vi "ke37xx Read Measurement Buffer.vi"(0 "VISA Resource Name":refnum<visa-resource-name>, 1 "Data To Read (All)":T1={"Readings"=TRUE, "Time Stamps"=TRUE, "Channels"=TRUE, "Units"=TRUE}, 5 "Buffer Name":string, 7 "Start Index (1)":i32=1 min=1, 9 "End Index (-1: Read All)":i32=-1 min=-1, 11 "error in (no error)":errorcluster, 12 "Time Stamp Format (0: UTC)":enum16{"UTC Time", "1588 Time"}(ring), 13 "Bytes To Read (1024)":u32=1024, 14 "Timeout (10 seconds)":u32=10000) -> (2 "Units":string[](array[string]), 3 "Channels":string[](array[string]), 4 "VISA Resource Name Out":refnum<visa-resource-name>, 6 "Readings":dbl[](array[numeric]) format="%#_6e", 8 "Time Stamps":cluster{"Seconds":u32, "Fraction":dbl}[](array[cluster]), 10 "Base Time Stamp":cluster{"Seconds":u32, "Fraction":dbl}, 15 "error out":errorcluster)   [LabVIEW 2009, in "Keithley 3700 Series.lvlib"]
doc: "This VI allows you to retrieve readings stored in a measurement buffer. You can optionally retrieve timestamp data, formatted readigns, measurement units, and channels measured."
uses:
  <instrlib>/Keithley 3706/Keithley 3700 Series.lvlib
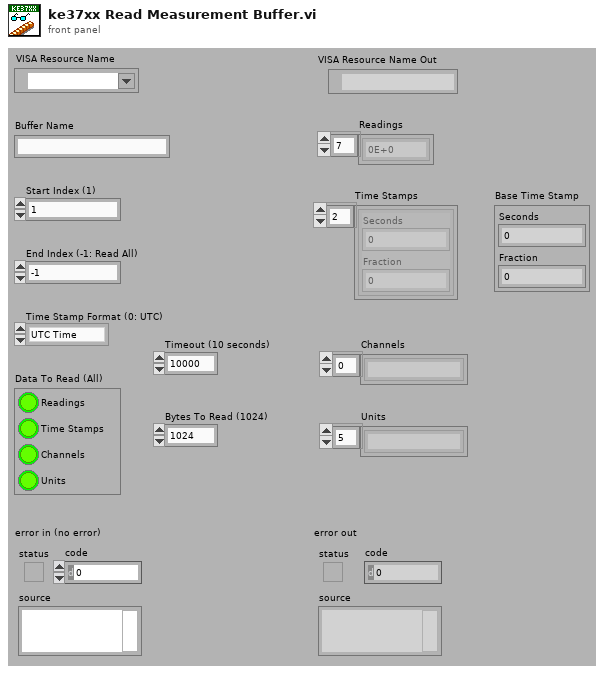
[diagram p1: front panel]
types:
  T1 = cluster{"Readings":bool, "Time Stamps":bool, "Channels":bool, "Units":bool}
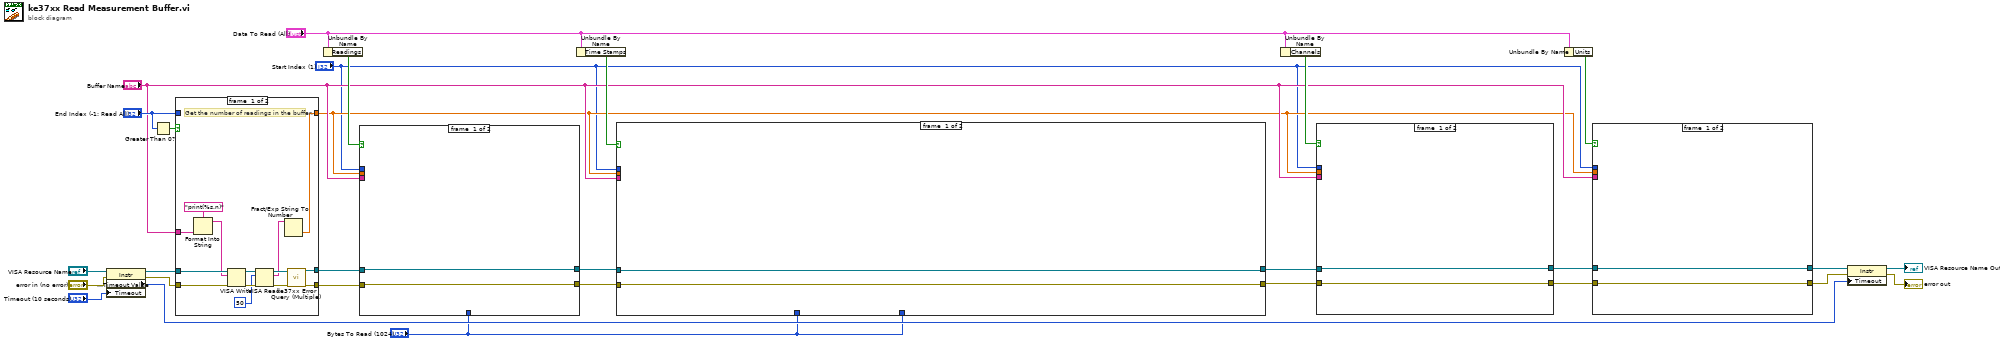
[diagram p0: block diagram]
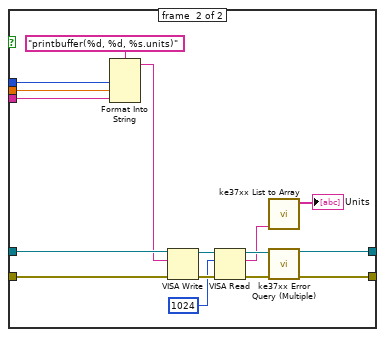
[diagram p2: hidden frame]
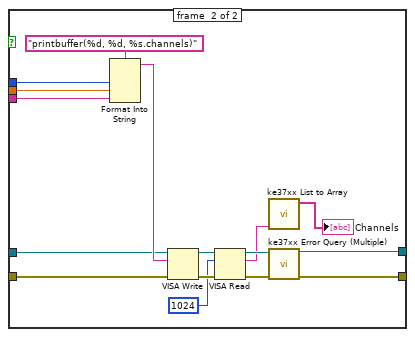
[diagram p3: hidden frame]
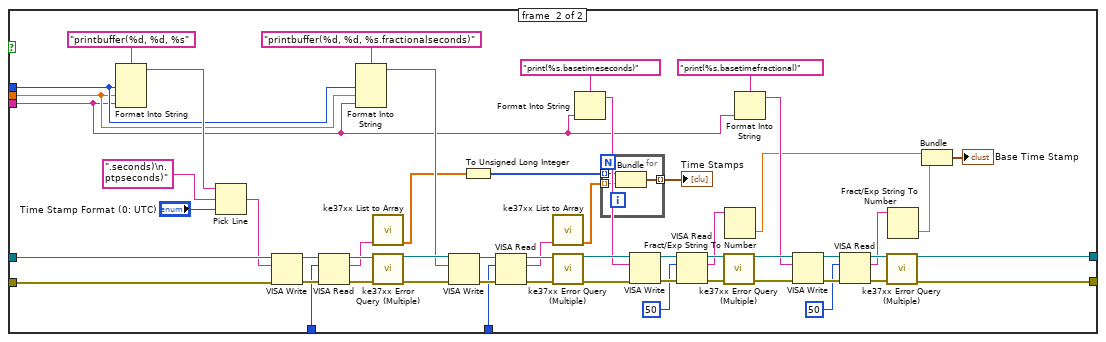
[diagram p4: hidden frame]
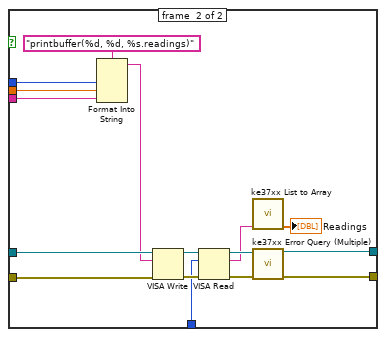
[diagram p5: hidden frame]
diagram:
  n1 = property class="Instr"(reference="VISA Resource Name", error in="error in (no error)", "Timeout"="Timeout (10 seconds)") -> (reference out=w12:refnum<visa-resource-name>, error out=w8:errorcluster, "General Settings:Timeout Value"=w2:u32)
  n2 = Greater Than 0?(x="End Index (-1: Read All)") -> (x > 0?=w29:bool)
  n3 = case shown="False" w29 {
    tunnel: w12 -> [w43 w45]
    tunnel: w8 -> [w42 w44]
    tunnel: [w41 w45] -> w28
    tunnel: [w40 w44] -> w27
    tunnel: "End Index (-1: Read All)" -> [_ w46]
    tunnel: [w31 w46] -> w15
    tunnel: "Buffer Name" -> [w30 _]
    frame #0 {
      # "Get the number of readings in the buffer."
      n4 = Format Into String(format string="print(%s.n)", w30) -> (resulting string=w38:string)  [unwired: 2 in, 1 out]
      n5 = VISA Write(VISA resource name=w43, write buffer=w38, error in (no error)=w42) -> (VISA resource name out=w37:refnum<visa-resource-name>, error out=w35:errorcluster)  [unwired: 1 out]
      n6 = VISA Read(VISA resource name=w37, byte count=u32 50, error in (no error)=w35) -> (VISA resource name out=w36:refnum<visa-resource-name>, read buffer=w32:string, error out=w34:errorcluster)  [unwired: 1 out]
      n7 = Fract/Exp String To Number(string=w32) -> (number=w31:dbl)  [unwired: 4 out]
      n8 = call <instrlib>:"ke37xx Error Query (Multiple).vi"("VISA resource name"=w36, "error in (no error)"=w34) -> ("VISA resource name out"=w41:refnum<visa-resource-name>, "error out"=w40:errorcluster)  [unwired: 12 out]
    }
    frame #1 {
    }
  }
  n9 = Unbundle By Name("Data To Read (All)") -> ("Readings"=w26:bool)
  n10 = case shown="True" w26 {
    tunnel: "Start Index (1)" -> [_ w62]
    tunnel: w28 -> [w48 w58]
    tunnel: w27 -> [w47 w57]
    tunnel: [w48 w56] -> w25
    tunnel: [w47 w55] -> w24
    tunnel: w15 -> [_ w52]
    tunnel: "Buffer Name" -> [_ w51]
    tunnel: "Bytes To Read (1024)" -> [_ w49]
    frame #0 {
    }
    frame #1 {
      n11 = Format Into String(format string="printbuffer(%d, %d, %s.readings)", w62, w52, w51) -> (resulting string=w54:string)  [unwired: 2 in, 1 out]
      n12 = VISA Write(VISA resource name=w58, write buffer=w54, error in (no error)=w57) -> (VISA resource name out=w59:refnum<visa-resource-name>, error out=w64:errorcluster)  [unwired: 1 out]
      n13 = VISA Read(VISA resource name=w59, byte count=w49, error in (no error)=w64) -> (VISA resource name out=w60:refnum<visa-resource-name>, read buffer=w50:string, error out=w61:errorcluster)  [unwired: 1 out]
      n14 = call <instrlib>:"ke37xx List to Array.vi"("List"=w50) -> ("Output Number Array"=→"Readings":dbl[])  [unwired: 1 in, 5 out]
      n15 = call <instrlib>:"ke37xx Error Query (Multiple).vi"("VISA resource name"=w60, "error in (no error)"=w61) -> ("VISA resource name out"=w56:refnum<visa-resource-name>, "error out"=w55:errorcluster)  [unwired: 12 out]
    }
  }
  n16 = Unbundle By Name("Data To Read (All)") -> ("Time Stamps"=w23:bool)
  n17 = case shown="True" w23 {
    tunnel: "Start Index (1)" -> [_ w104]
    tunnel: w25 -> [w66 w115]
    tunnel: w24 -> [w65 w114]
    tunnel: w15 -> [_ w103]
    tunnel: "Buffer Name" -> [_ w88]
    tunnel: [w66 w79] -> w11
    tunnel: [w65 w78] -> w10
    tunnel: "Bytes To Read (1024)" -> [_ w68]
    tunnel: "Bytes To Read (1024)" -> [_ w67]
    frame #0 {
    }
    frame #1 {
      n18 = Format Into String(format string="printbuffer(%d, %d, %s", w104, w103, w88) -> (resulting string=w111:string)  [unwired: 2 in, 1 out]
      n19 = Pick Line(string ("")=w111, multi-line string=".seconds)\n.ptpseconds)", line index="Time Stamp Format (0: UTC)") -> (output string=w110:string)
      n20 = VISA Write(VISA resource name=w115, write buffer=w110, error in (no error)=w114) -> (VISA resource name out=w116:refnum<visa-resource-name>, error out=w120:errorcluster)  [unwired: 1 out]
      n21 = VISA Read(VISA resource name=w116, byte count=w68, error in (no error)=w120) -> (VISA resource name out=w117:refnum<visa-resource-name>, read buffer=w77:string, error out=w118:errorcluster)  [unwired: 1 out]
      n22 = Format Into String(format string="printbuffer(%d, %d, %s.fractionalseconds)", w104, w103, w88) -> (resulting string=w102:string)  [unwired: 2 in, 1 out]
      n23 = call <instrlib>:"ke37xx List to Array.vi"("List"=w77) -> ("Output Number Array"=w72:dbl[])  [unwired: 1 in, 5 out]
      n24 = call <instrlib>:"ke37xx Error Query (Multiple).vi"("VISA resource name"=w117, "error in (no error)"=w118) -> ("VISA resource name out"=w107:refnum<visa-resource-name>, "error out"=w106:errorcluster)  [unwired: 12 out]
      n25 = VISA Write(VISA resource name=w107, write buffer=w102, error in (no error)=w106) -> (VISA resource name out=w109:refnum<visa-resource-name>, error out=w108:errorcluster)  [unwired: 1 out]
      n26 = To Unsigned Long Integer(number=w72) -> (unsigned 32bit integer=w71:u32[])
      n27 = VISA Read(VISA resource name=w109, byte count=w67, error in (no error)=w108) -> (VISA resource name out=w96:refnum<visa-resource-name>, read buffer=w76:string, error out=w95:errorcluster)  [unwired: 1 out]
      n28 = call <instrlib>:"ke37xx List to Array.vi"("List"=w76) -> ("Output Number Array"=w70:dbl[])  [unwired: 1 in, 5 out]
      n29 = call <instrlib>:"ke37xx Error Query (Multiple).vi"("VISA resource name"=w96, "error in (no error)"=w95) -> ("VISA resource name out"=w94:refnum<visa-resource-name>, "error out"=w93:errorcluster)  [unwired: 12 out]
      n30 = Format Into String(format string="print(%s.basetimeseconds)", w88) -> (resulting string=w90:string)  [unwired: 2 in, 1 out]
      n31 = for {
        tunnel: w71 -> [w124] mode=indexing
        tunnel: w70 -> [w123] mode=indexing
        tunnel: [w122] -> w69 mode=indexing
        n32 = Bundle(w124, w123) -> (w122:cluster{u32, dbl})  [unwired: 1 out]
      }
      "Time Stamps" <- w69
      n33 = VISA Write(VISA resource name=w94, write buffer=w90, error in (no error)=w93) -> (VISA resource name out=w99:refnum<visa-resource-name>, error out=w101:errorcluster)  [unwired: 1 out]
      n34 = VISA Read(VISA resource name=w99, byte count=u32 50, error in (no error)=w101) -> (VISA resource name out=w92:refnum<visa-resource-name>, read buffer=w89:string, error out=w91:errorcluster)  [unwired: 1 out]
      n35 = call <instrlib>:"ke37xx Error Query (Multiple).vi"("VISA resource name"=w92, "error in (no error)"=w91) -> ("VISA resource name out"=w83:refnum<visa-resource-name>, "error out"=w82:errorcluster)  [unwired: 12 out]
      n36 = Fract/Exp String To Number(string=w89) -> (number=w75:dbl)  [unwired: 1 in, 3 out]
      n37 = Format Into String(format string="print(%s.basetimefractional)", w88) -> (resulting string=w81:string)  [unwired: 2 in, 1 out]
      n38 = VISA Write(VISA resource name=w83, write buffer=w81, error in (no error)=w82) -> (VISA resource name out=w85:refnum<visa-resource-name>, error out=w121:errorcluster)  [unwired: 1 out]
      n39 = VISA Read(VISA resource name=w85, byte count=u32 50, error in (no error)=w121) -> (VISA resource name out=w86:refnum<visa-resource-name>, read buffer=w80:string, error out=w87:errorcluster)  [unwired: 1 out]
      n40 = call <instrlib>:"ke37xx Error Query (Multiple).vi"("VISA resource name"=w86, "error in (no error)"=w87) -> ("VISA resource name out"=w79:refnum<visa-resource-name>, "error out"=w78:errorcluster)  [unwired: 12 out]
      n41 = Fract/Exp String To Number(string=w80) -> (number=w74:dbl)  [unwired: 4 out]
      n42 = Bundle(w75, w74) -> (→"Base Time Stamp":cluster{dbl, dbl})  [unwired: 1 out]
    }
  }
  n43 = Unbundle By Name("Data To Read (All)") -> ("Channels"=w21:bool)
  n44 = case shown="True" w21 {
    tunnel: "Start Index (1)" -> [_ w140]
    tunnel: [w126 w135] -> w20
    tunnel: [w125 w134] -> w19
    tunnel: w15 -> [_ w132]
    tunnel: "Buffer Name" -> [_ w131]
    tunnel: w11 -> [w126 w129]
    tunnel: w10 -> [w125 w128]
    frame #0 {
    }
    frame #1 {
      n45 = Format Into String(format string="printbuffer(%d, %d, %s.channels)", w140, w132, w131) -> (resulting string=w133:string)  [unwired: 2 in, 1 out]
      n46 = VISA Write(VISA resource name=w129, write buffer=w133, error in (no error)=w128) -> (VISA resource name out=w136:refnum<visa-resource-name>, error out=w142:errorcluster)  [unwired: 1 out]
      n47 = VISA Read(VISA resource name=w136, byte count=u32 1024, error in (no error)=w142) -> (VISA resource name out=w137:refnum<visa-resource-name>, read buffer=w130:string, error out=w138:errorcluster)  [unwired: 1 out]
      n48 = call <instrlib>:"ke37xx List to Array.vi"("List"=w130) -> ("Output String Array"=→"Channels":string[])  [unwired: 1 in, 5 out]
      n49 = call <instrlib>:"ke37xx Error Query (Multiple).vi"("VISA resource name"=w137, "error in (no error)"=w138) -> ("VISA resource name out"=w135:refnum<visa-resource-name>, "error out"=w134:errorcluster)  [unwired: 12 out]
    }
  }
  n50 = Unbundle By Name("Data To Read (All)") -> ("Units"=w17:bool)
  n51 = case shown="True" w17 {
    tunnel: [w144 w153] -> w6
    tunnel: [w143 w152] -> w4
    tunnel: w20 -> [w144 w160]
    tunnel: w19 -> [w143 w150]
    tunnel: "Buffer Name" -> [_ w149]
    tunnel: w15 -> [_ w148]
    tunnel: "Start Index (1)" -> [_ w147]
    frame #0 {
    }
    frame #1 {
      n52 = Format Into String(format string="printbuffer(%d, %d, %s.units)", w147, w148, w149) -> (resulting string=w151:string)  [unwired: 2 in, 1 out]
      n53 = VISA Write(VISA resource name=w160, write buffer=w151, error in (no error)=w150) -> (VISA resource name out=w154:refnum<visa-resource-name>, error out=w159:errorcluster)  [unwired: 1 out]
      n54 = VISA Read(VISA resource name=w154, byte count=u32 1024, error in (no error)=w159) -> (VISA resource name out=w155:refnum<visa-resource-name>, read buffer=w146:string, error out=w156:errorcluster)  [unwired: 1 out]
      n55 = call <instrlib>:"ke37xx List to Array.vi"("List"=w146) -> ("Output String Array"=→"Units":string[])  [unwired: 1 in, 5 out]
      n56 = call <instrlib>:"ke37xx Error Query (Multiple).vi"("VISA resource name"=w155, "error in (no error)"=w156) -> ("VISA resource name out"=w153:refnum<visa-resource-name>, "error out"=w152:errorcluster)  [unwired: 12 out]
    }
  }
  n57 = property class="Instr"(reference=w6, error in=w4, "Timeout"=w2) -> (reference out=→"VISA Resource Name Out":refnum<visa-resource-name>, error out=→"error out":errorcluster)
